vi "TestRecordGeneratingLabVIEWPython.vi"() -> ()   [LabVIEW 2018]
uses:
  <vilib>/Enthought/Python Integration Toolkit/Python Integration Toolkit.lvlib
panel:
  in  "Result File Name (must include .xlsx)":string
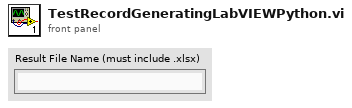
[diagram p1: front panel]
types:
  T1 = typedef "Python Integration Toolkit.lvlib/Session ID.ctl" = u64
  T2 = typedef "Python Integration Toolkit.lvlib/Python Objects.ctl" = variant
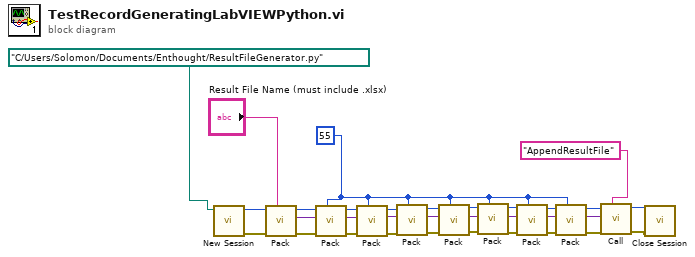
[diagram p0: block diagram]
diagram:
  w1 = 55
  n1 = call <vilib>:"New Session.vi"("Path to Python Module (.py File)"=path "C:/Users/Solomon/Documents/Enthought/ResultFileGenerator.py") -> ("error out"=w31:errorcluster, "Session ID out"=w32:T1)  [unwired: 9 in]
  n2 = call <vilib>:"Pack.vi"("Argument"="Result File Name (must include .xlsx)", "error in (no error)"=w31, "Session ID"=w32) -> ("error out"=w29:errorcluster, "Python Object References Out"=w28:T2, "Session ID out"=w30:T1)  [unwired: 6 in]
  n3 = call <vilib>:"Pack.vi"("Argument"=w1, "error in (no error)"=w29, "Python Object References In"=w28, "Session ID"=w30) -> ("error out"=w23:errorcluster, "Python Object References Out"=w24:T2, "Session ID out"=w25:T1)  [unwired: 5 in]
  n4 = call <vilib>:"Pack.vi"("Argument"=w1, "error in (no error)"=w23, "Python Object References In"=w24, "Session ID"=w25) -> ("error out"=w20:errorcluster, "Python Object References Out"=w21:T2, "Session ID out"=w22:T1)  [unwired: 5 in]
  n5 = call <vilib>:"Pack.vi"("Argument"=w1, "error in (no error)"=w20, "Python Object References In"=w21, "Session ID"=w22) -> ("error out"=w17:errorcluster, "Python Object References Out"=w18:T2, "Session ID out"=w19:T1)  [unwired: 5 in]
  n6 = call <vilib>:"Pack.vi"("Argument"=w1, "error in (no error)"=w17, "Python Object References In"=w18, "Session ID"=w19) -> ("error out"=w14:errorcluster, "Python Object References Out"=w15:T2, "Session ID out"=w16:T1)  [unwired: 5 in]
  n7 = call <vilib>:"Pack.vi"("Argument"=w1, "error in (no error)"=w14, "Python Object References In"=w15, "Session ID"=w16) -> ("error out"=w11:errorcluster, "Python Object References Out"=w12:T2, "Session ID out"=w13:T1)  [unwired: 5 in]
  n8 = call <vilib>:"Pack.vi"("Argument"=w1, "error in (no error)"=w11, "Python Object References In"=w12, "Session ID"=w13) -> ("error out"=w8:errorcluster, "Python Object References Out"=w9:T2, "Session ID out"=w10:T1)  [unwired: 5 in]
  n9 = call <vilib>:"Pack.vi"("Argument"=w1, "error in (no error)"=w8, "Python Object References In"=w9, "Session ID"=w10) -> ("error out"=w5:errorcluster, "Python Object References Out"=w6:T2, "Session ID out"=w7:T1)  [unwired: 5 in]
  n10 = call <vilib>:"Call.vi"("Function or Method Name"="AppendResultFile" ("Function Name"), "error in (no error)"=w5, "Python Object References In"=w6, "Session ID"=w7) -> ("error out"=w26:errorcluster, "Session ID out"=w27:T1)  [unwired: 5 in, 1 out]
  n11 = call <vilib>:"Close Session.vi"("error in (no error)"=w26, "Session ID"=w27) -> ()  [unwired: 9 in, 1 out]
